vi "Test Controller.vi"   [LabVIEW 2020]
uses:
  Controller/Controller/Controller/Controller.lvclass
  C:/Program Files (x86)/National Instruments/LabVIEW 2020/vi.lib/ActorFramework/Actor/Actor.lvclass
  <vilib>/ActorFramework/Actor/Actor.lvclass
types:
  T1 = enum32{"Invalid", "Standard", "Closed", "Hidden", "Minimized", "Maximized"}
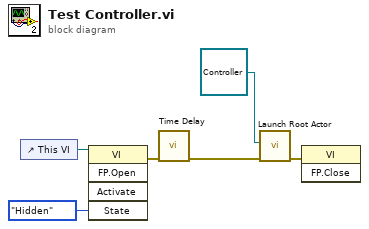
[diagram p0: block diagram]
diagram:
  n1 = control-ref of="This VI"() -> (w3:refnum<vi>)
  n2 = invoke class="VI" method="FP.Open"(reference=w3, "State"=T1."Hidden") -> (error out=w2:errorcluster)  [unwired: 3 in, 4 out]
  n3 = call "Time Delay"("error in (no error)"=w2) -> ("error out"=w1:errorcluster)  [unwired: 10 in]
  n4 = call <vilib>:"Launch Root Actor.vi"("error in (no error)"=w1, "Actor"=refnum<class "Controller.lvclass"> refnum ("Controller.lvlib:Controller.lvclass")) -> ("error out"=w5:errorcluster)  [unwired: 8 in, 1 out]
  n5 = invoke class="VI" method="FP.Close"(error in=w5) -> ()  [unwired: 2 in, 3 out]
